vi "Write.vi"(8 "error in (no error)":errorcluster, 9 "Variant":variant, 10 "String":string, 11 "UDP in":refnum<class "UDP.lvclass">) -> (0 "error out":errorcluster, 3 "UDP out":refnum<class "UDP.lvclass">)   [LabVIEW 2013, in "Protocol Classes.lvlib" / "UDP.lvclass"]
uses:
  UDP.lvclass
  UDP.lvclass/UDP.ctl
  Data Access/Read Target Port.vi
  Data Access/Read Target IP Address.vi
  Data Access/Read UDP Ref.vi
  Data Access/Write UDP Ref.vi
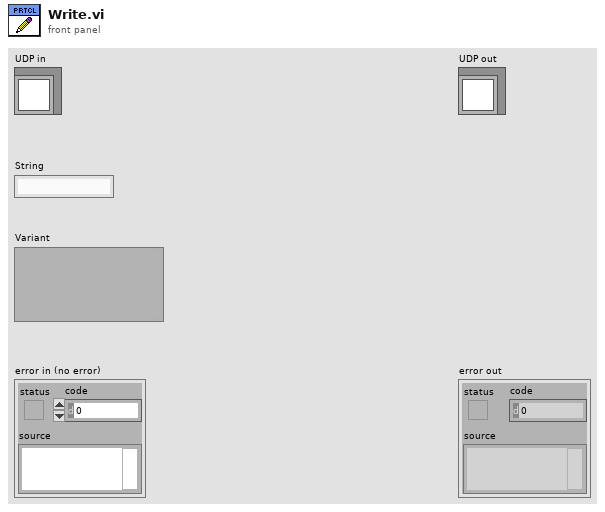
[diagram p1: front panel]
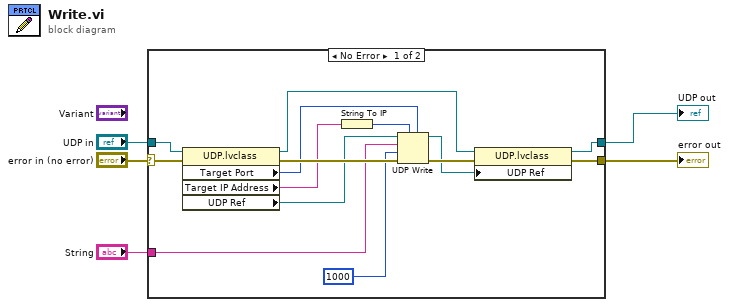
[diagram p0: block diagram]
diagram:
  n1 = case shown="No Error" "error in (no error)" {
    selector: "error in (no error)" -> [w11 w21]
    tunnel: "UDP in" -> [w18 w20]
    tunnel: [w14 w21] -> w5
    tunnel: [w13 w20] -> w4
    tunnel: "String" -> [w12 _]
    frame No Error {
      n2 = property class="UDP.lvclass"(reference=w18, error in=w11) -> (reference out=w16:refnum<class "UDP.lvclass">, error out=w19:errorcluster, "Target Port"=w9:u16, "Target IP Address"=w8:string, "UDP Ref"=w6:refnum<k16>)
      n3 = String To IP(1:w8) -> (0:w7:u32)
      n4 = UDP Write(address=w7, port or service name=w9, connection ID=w6, data in=w12, 8:w19, 9:1000 ("timeout ms (25000)")) -> (error out=w17:errorcluster, 3:w15:refnum<k16>)
      n5 = property class="UDP.lvclass"(reference=w16, error in=w17, "UDP Ref"=w15) -> (reference out=w13:refnum<class "UDP.lvclass">, error out=w14:errorcluster)
    }
    frame Error {
    }
  }
  "error out" <- w5
  "UDP out" <- w4
